vi "phase_maps_to_pixel_difference_float.vi"(10 "dist phase map":dbl[][](array[numeric]), 11 "oirg phase map":dbl[][](array[numeric])) -> (3 "displacement map":i32[][](array[numeric]))   [LabVIEW 2011]
doc: "The input array must be unwrapped phase maps, that are normalize to the same span (i.e. 0 to 255) and where the masked pixels are 0."
uses:
  global_vars.vi
panel:
  out "input":dbl[][](graph)
  in  "dbl_pxar_orig_unwrap":dbl[][](array[numeric])=array1050x1050[1102500 elements]
  in  "dbl_pxar_dist_unwrap":dbl[][](array[numeric])=array1050x1050[1102500 elements]
  in  "Stop":bool
  out "displacement":i32[](graph)
  in  "row":i32(slide) scale=0.0..1000.0
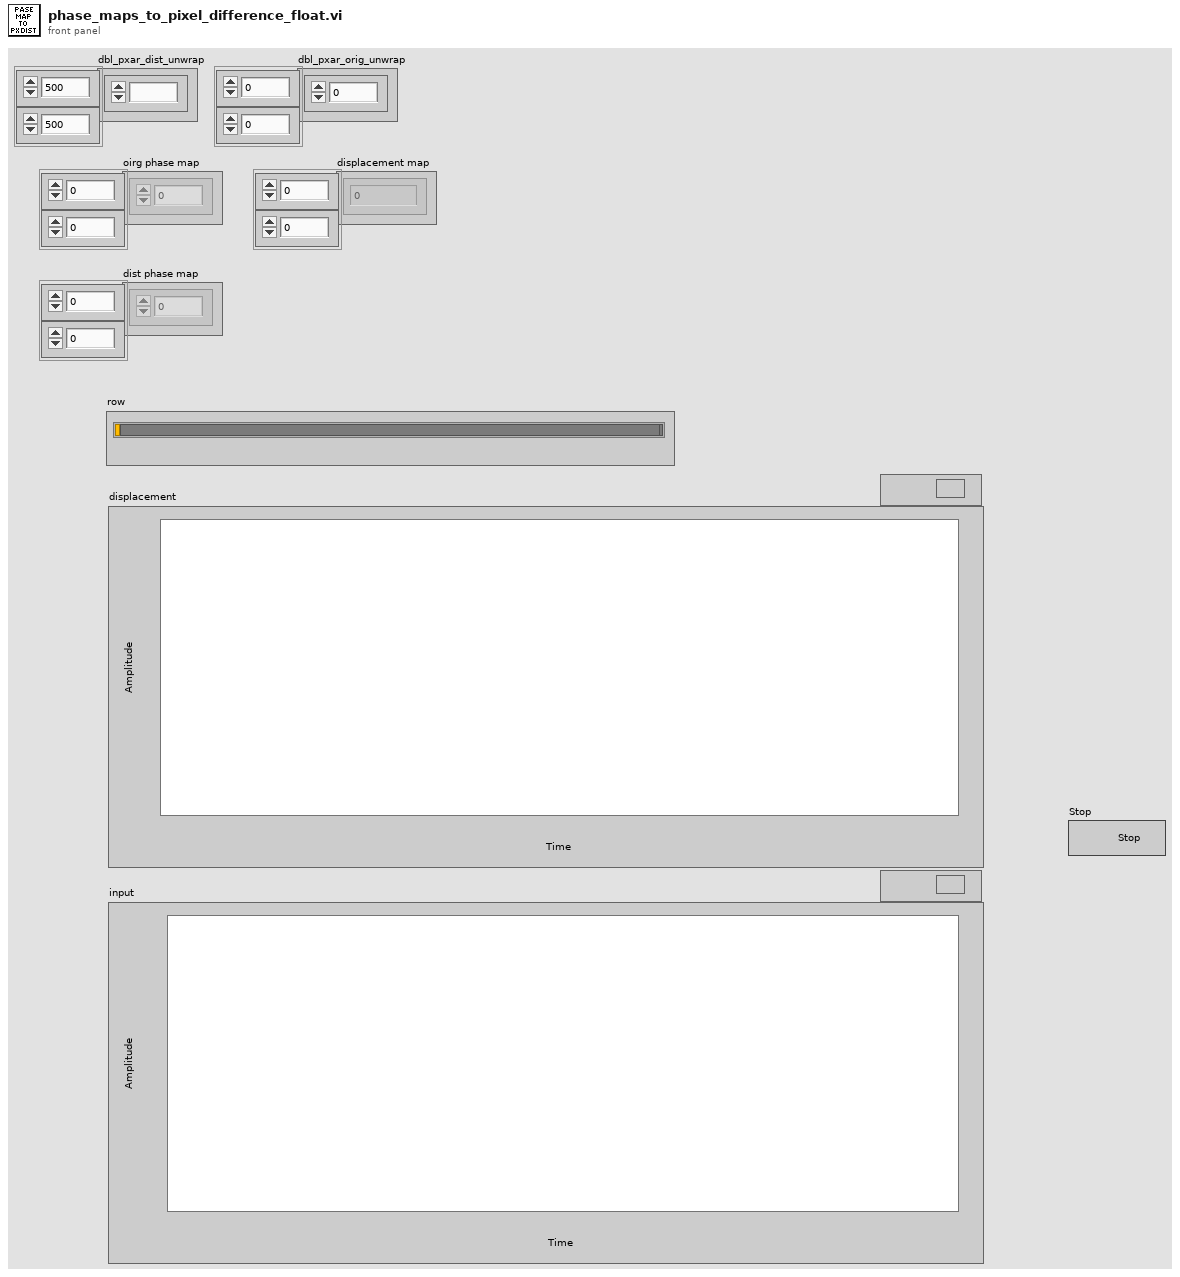
[diagram p1: front panel]
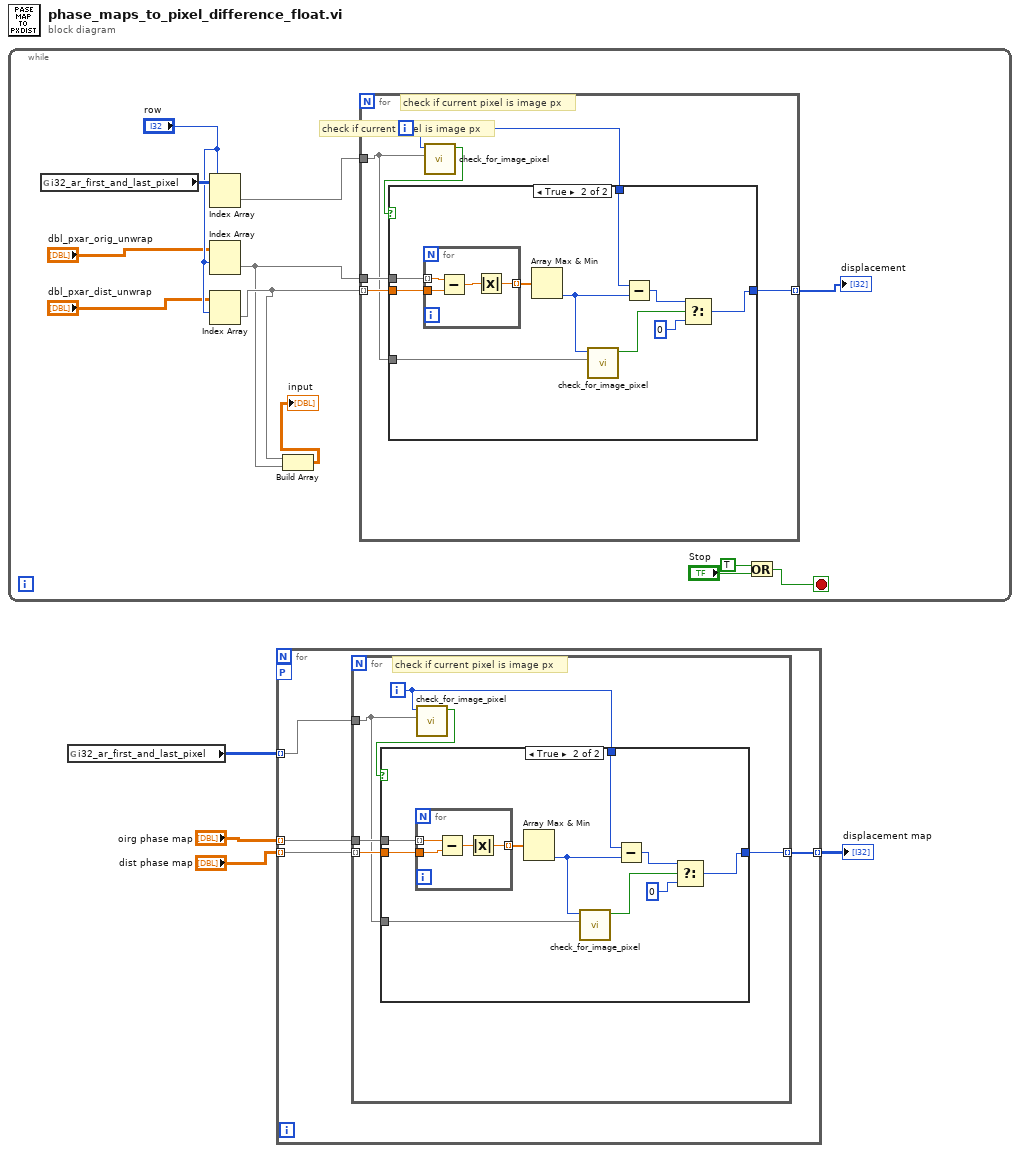
[diagram p0: block diagram]
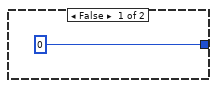
[diagram p2: hidden frame]
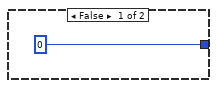
[diagram p3: hidden frame]
diagram:
  n1 = while {
    stop <- w13 stop-if-true
    # "check if current pixel is image px"
    n2 = global read "global_vars.vi" "i32_ar_first_and_last_pixel"() -> (w16:i32[][])
    n3 = Index Array(array=w16, index (row)="row") -> (element=w14:i32[])  [unwired: 1 in]
    n4 = Index Array(array="dbl_pxar_orig_unwrap", index (row)="row") -> (element=w6:dbl[])  [unwired: 1 in]
    n5 = Index Array(array="dbl_pxar_dist_unwrap", index (row)="row") -> (element=w7:dbl[])  [unwired: 1 in]
    n6 = Build Array(w7, w6) -> (→"input":dbl[][])
    n7 = for {
      tunnel: w7 -> [w22] mode=indexing
      tunnel: [w21] -> w8 mode=indexing
      tunnel: w6 -> [w20]
      tunnel: w14 -> [w17]
      i -> [w18]
      # "check if current pixel is image px"
      n8 = call "check_for_image_pixel.vi"("i32_ar_first_and_last_pixel"=w17, "current index"=w18) -> ("image pixel"=w19:bool)  [unwired: 9 in]
      n9 = case shown="True" w19 {
        tunnel: w22 -> [_ w33]
        tunnel: [0 w28] -> w21
        tunnel: w20 -> [_ w31]
        tunnel: w18 -> [_ w30]
        tunnel: w17 -> [_ w27]
        frame False {
        }
        frame True {
          n10 = for {
            tunnel: w31 -> [w37] mode=indexing
            tunnel: w33 -> [w36]
            tunnel: [w35] -> w32 mode=indexing
            n11 = Subtract(x=w37, y=w36) -> (x-y=w34:dbl)
            n12 = Absolute Value(x=w34) -> (abs(x)=w35:dbl)
          }
          n13 = Array Max & Min(array=w32) -> (min index (indices)=w26:i32)  [unwired: 3 out]
          n14 = call "check_for_image_pixel.vi"("i32_ar_first_and_last_pixel"=w27, "current index"=w26) -> ("image pixel"=w25:bool)  [unwired: 9 in]
          n15 = Subtract(x=w30, y=w26) -> (x-y=w29:i32)
          n16 = Select(t=w29, s=w25, f=0) -> (s? t:f=w28:i32)
        }
      }
    }
    "displacement" <- w8
    n17 = Or(x=TRUE, y="Stop") -> (x .or. y?=w13:bool)
  }
  n18 = global read "global_vars.vi" "i32_ar_first_and_last_pixel"() -> (w1:i32[][])
  n19 = for {
    tunnel: "dist phase map" -> [w41] mode=indexing
    tunnel: "oirg phase map" -> [w40] mode=indexing
    workers-P: _ -> [_]
    tunnel: [w39] -> w4 mode=indexing
    tunnel: w1 -> [w38] mode=indexing
    n20 = for {
      tunnel: w41 -> [w47] mode=indexing
      tunnel: [w46] -> w39 mode=indexing
      tunnel: w40 -> [w45]
      tunnel: w38 -> [w42]
      i -> [w43]
      # "check if current pixel is image px"
      n21 = call "check_for_image_pixel.vi"("i32_ar_first_and_last_pixel"=w42, "current index"=w43) -> ("image pixel"=w44:bool)  [unwired: 9 in]
      n22 = case shown="True" w44 {
        tunnel: w47 -> [_ w58]
        tunnel: [0 w53] -> w46
        tunnel: w45 -> [_ w56]
        tunnel: w43 -> [_ w55]
        tunnel: w42 -> [_ w52]
        frame False {
        }
        frame True {
          n23 = for {
            tunnel: w56 -> [w62] mode=indexing
            tunnel: w58 -> [w61]
            tunnel: [w60] -> w57 mode=indexing
            n24 = Subtract(x=w62, y=w61) -> (x-y=w59:dbl)
            n25 = Absolute Value(x=w59) -> (abs(x)=w60:dbl)
          }
          n26 = Array Max & Min(array=w57) -> (min index (indices)=w51:i32)  [unwired: 3 out]
          n27 = call "check_for_image_pixel.vi"("i32_ar_first_and_last_pixel"=w52, "current index"=w51) -> ("image pixel"=w50:bool)  [unwired: 9 in]
          n28 = Subtract(x=w55, y=w51) -> (x-y=w54:i32)
          n29 = Select(t=w54, s=w50, f=0) -> (s? t:f=w53:i32)
        }
      }
    }
  }
  "displacement map" <- w4
